vi "Update Binaries.vi"() -> ()   [LabVIEW 2011]
panel:
  out "Copied dll Files":string
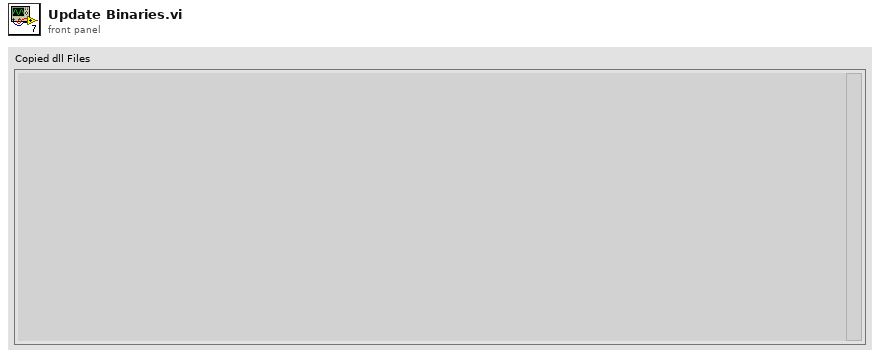
[diagram p1: front panel]
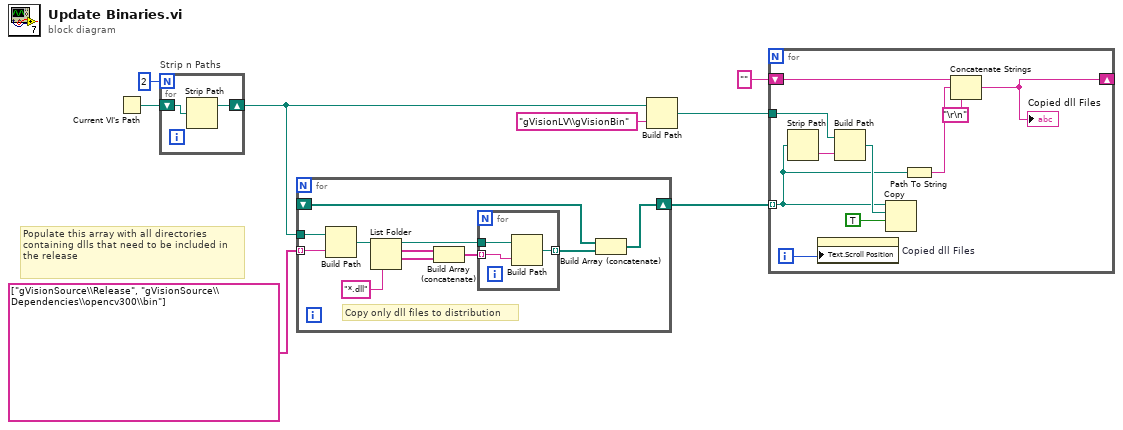
[diagram p0: block diagram]
diagram:
  # "Populate this array with all directories containing dlls that need to be included in the release"
  n1 = Current VI's Path() -> (path=w8:path)
  n2 = for "Strip n Paths" {
    N: 2 -> [_]
    shift-right: [w9] -> w3
    shift-left: w8 -> [w10]
    n3 = Strip Path(path=w10) -> (stripped path=w9:path)  [unwired: 1 out]
  }
  n4 = for {
    tunnel: w3 -> [w15]
    tunnel: string[] ["gVisionSource\\Release", "gVisionSource\\Dependencies\\opencv300\\bin"] -> [w14] mode=indexing
    shift-right: [w13] -> w1
    shift-left: _ -> [w12]
    # "Copy only dll files to distribution"
    n5 = Build Path(base path=w15, name or relative path=w14) -> (appended path=w21:path)
    n6 = List Folder(path=w21, pattern="*.dll") -> (path out=w17:path, filenames=w20:string[], folder names=w19:string[])  [unwired: 2 in, 1 out]
    n7 = Build Array (concatenate)(w20, w19) -> (w18:string[])
    n8 = for {
      tunnel: w18 -> [w24] mode=indexing
      tunnel: w17 -> [w23]
      tunnel: [w22] -> w11 mode=indexing
      n9 = Build Path(base path=w23, name or relative path=w24) -> (appended path=w22:path)
    }
    n10 = Build Array (concatenate)(w12, w11) -> (w13:path[])
  }
  n11 = Build Path(base path=w3, name or relative path="gVisionLV\\gVisionBin") -> (appended path=w5:path)
  n12 = for {
    tunnel: w1 -> [w30] mode=indexing
    tunnel: w5 -> [w33]
    shift-right: [w26] -> _
    shift-left: "" -> [w29]
    i -> [w25]
    n13 = Strip Path(path=w30) -> (name=w34:string)  [unwired: 1 out]
    n14 = property on="Copied dll Files" class="Str"("Text.Scroll Position"=w25) -> ()  [unwired: 2 in, 2 out]
    n15 = Build Path(base path=w33, name or relative path=w34) -> (appended path=w32:path)
    n16 = Copy(9:TRUE ("overwrite (F)"), 10:w32, 11:w30) -> ()  [unwired: 2 in, 3 out]
    n17 = Path To String(path=w30) -> (string=w28:string)
    n18 = Concatenate Strings(w29, w28, "\r\n") -> (w26:string)
    "Copied dll Files" <- w26
  }
